vi "DSC TSV to PGSQL.vi"() -> ()   [LabVIEW 2019]
uses:
  src/LV-Data.PG/LV-Data.PGSQL.lvclass
  1022e062-927a-46ce-8191-545f75b782fa.vi
  <vilib>/dlg_ctls.llb/Space Constant.vi
  src/LV-Data.PG/API/Write Variable (multirow).vi
  <vilib>/Utility/error.llb/Clear Errors.vi
  <userlib>/_OpenG.lib/file/file.llb/Build Path - File Names Array__ogtk.vi
  src/LV-Data.PG/Private/INSERT Multivalue.vi
  DSC TSV Process Path.vi
panel:
  in  "Process Files":bool
  in  "Load Translation":bool
  in  "Save Translation":bool
  in  "Get PGSQL":bool
  in  "List Files":bool
  in  "Macro":bool
  out "Status":string
  out "Processed Files":string
  out "Paths":string[][](table)
  in  "Instrument Path":path=path "G:/.shortcut-targets-by-id/1WDr4dR83sFDxMqrJrBnKdnzPXtLPCjmG/Database Data"
  in  "OK":bool
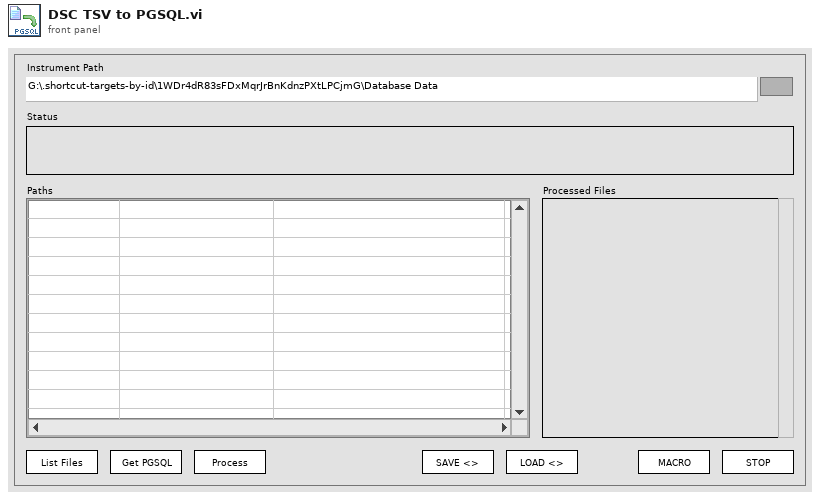
[diagram p1: front panel]
types:
  T1 = enum32{"Invalid", "Standard", "Closed", "Hidden", "Minimized", "Maximized"}
  T2 = enum32{"invalid app kind", "Development System", "Run Time System", "Student Edition", "Embedded LabVIEW", "Evaluation", "Custom"}
  T3 = cluster{"Core":cluster{"Current VI Reference":refnum<vi>, "Close Panel on Exit?":bool}, "Data.PG":refnum<class "LV-Data.PGSQL.lvclass">, "Instrument Path":path, "Variables":path[], "Files":path[][], "DSC Table":string[], "DSC Variable":string[], "DSC Units":string[], "PGSQL Paths":string[]}
  T4 = cluster{"Current VI Reference":refnum<vi>, "Close Panel on Exit?":bool}
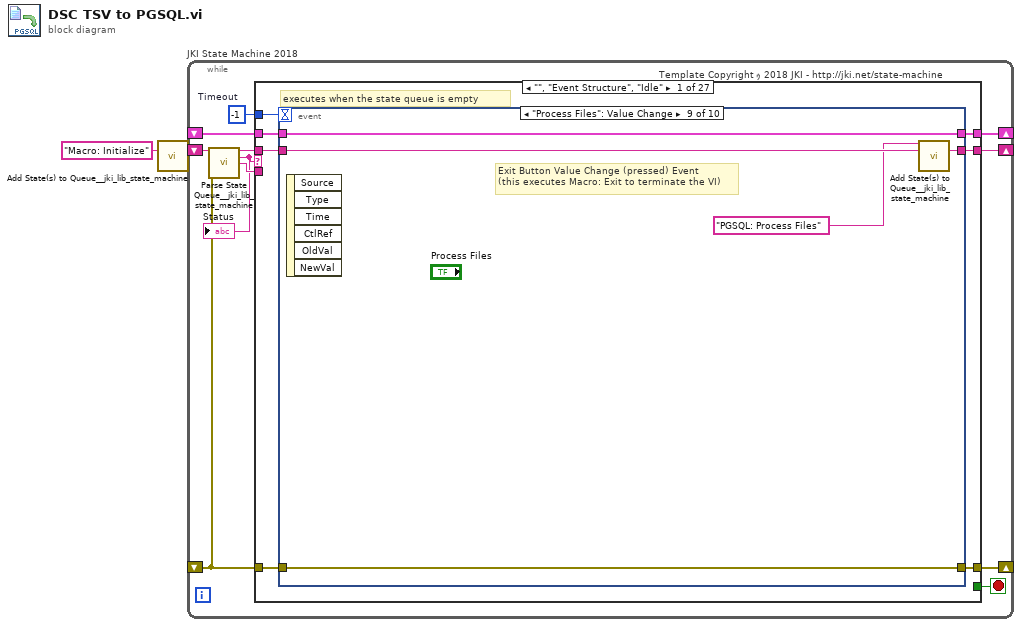
[diagram p0: block diagram]
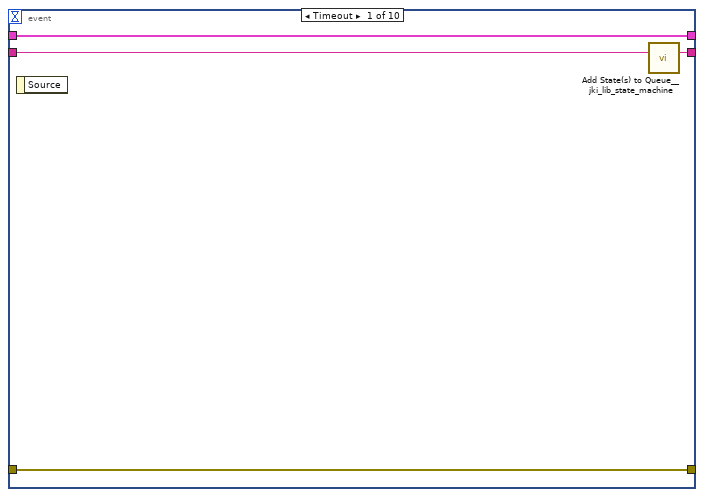
[diagram p2: hidden frame]
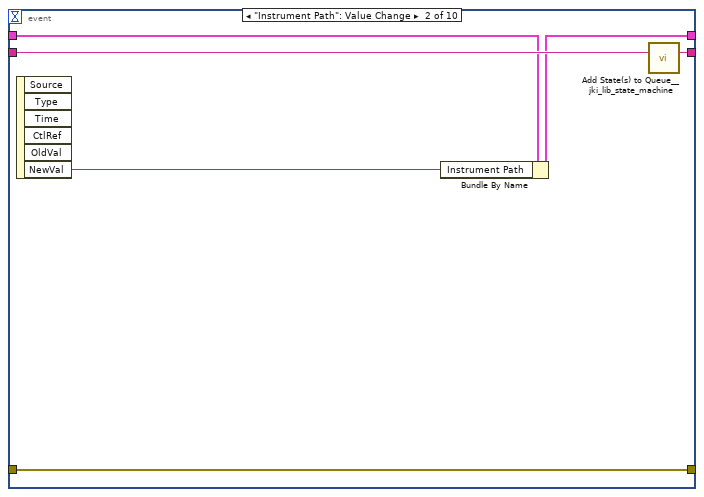
[diagram p3: hidden frame]
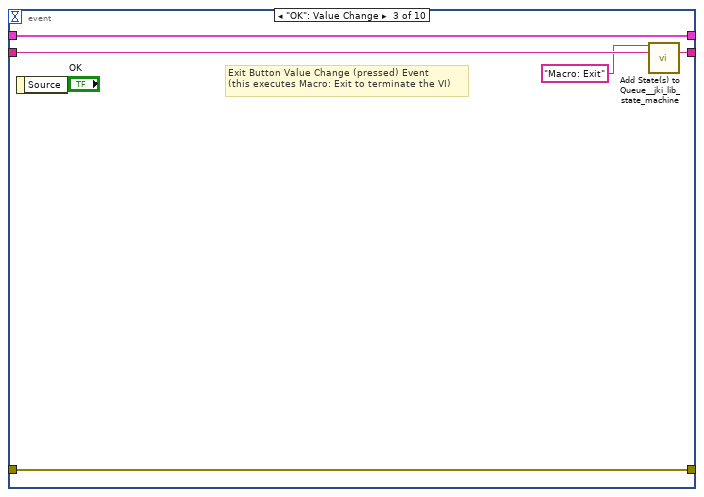
[diagram p4: hidden frame]
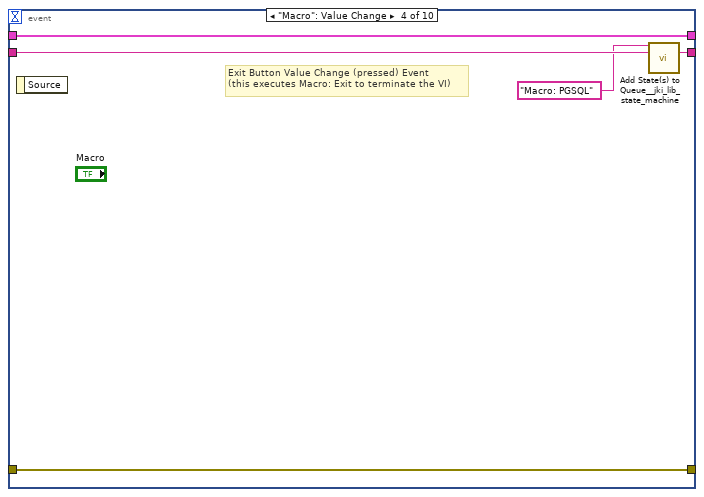
[diagram p5: hidden frame]
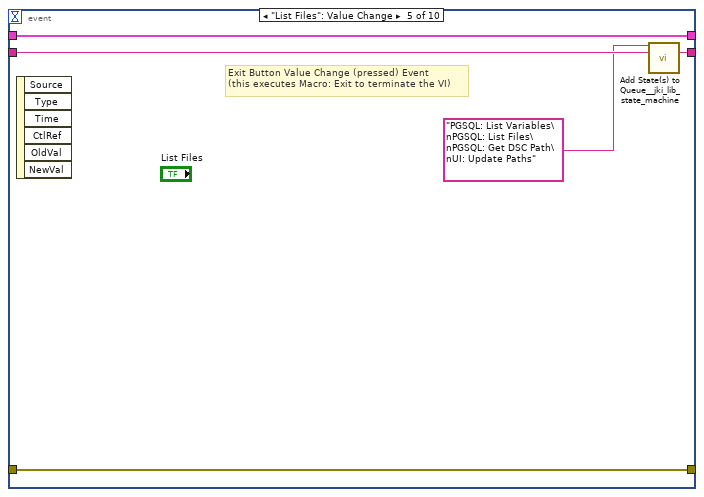
[diagram p6: hidden frame]
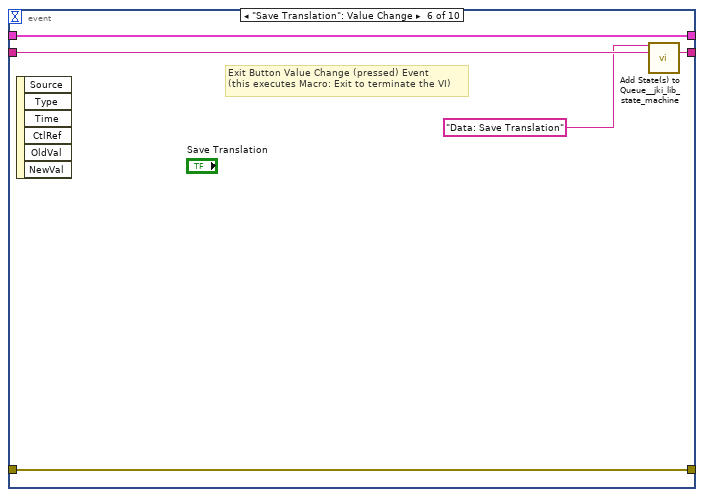
[diagram p7: hidden frame]
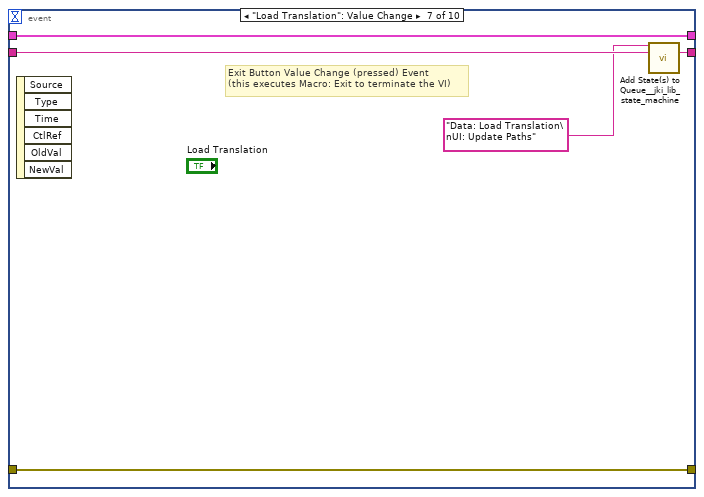
[diagram p8: hidden frame]
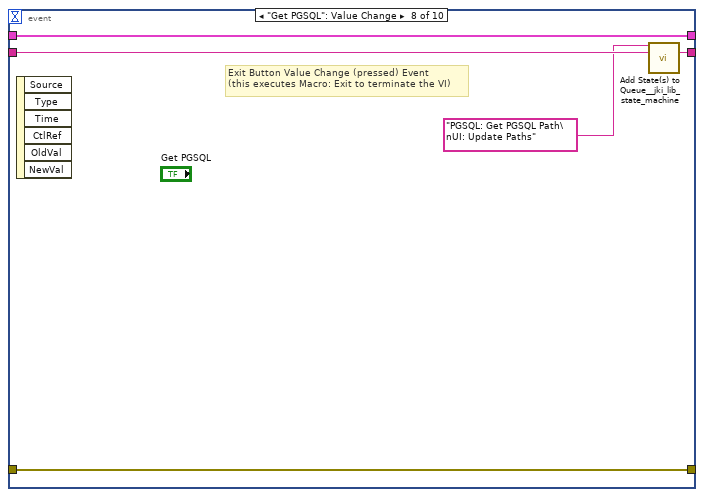
[diagram p9: hidden frame]
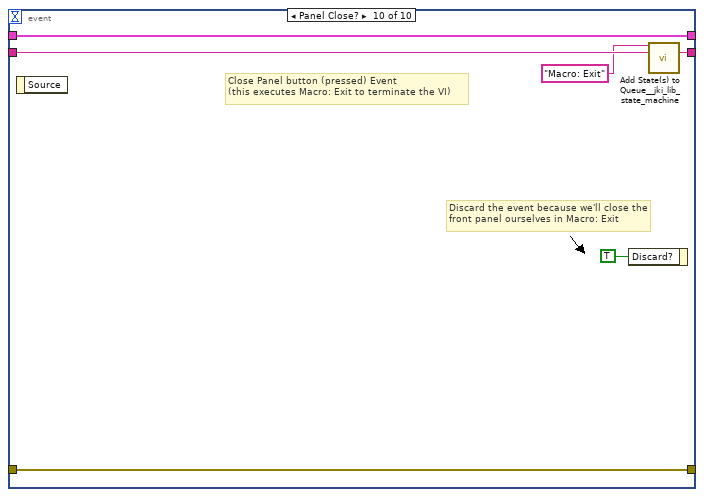
[diagram p10: hidden frame]
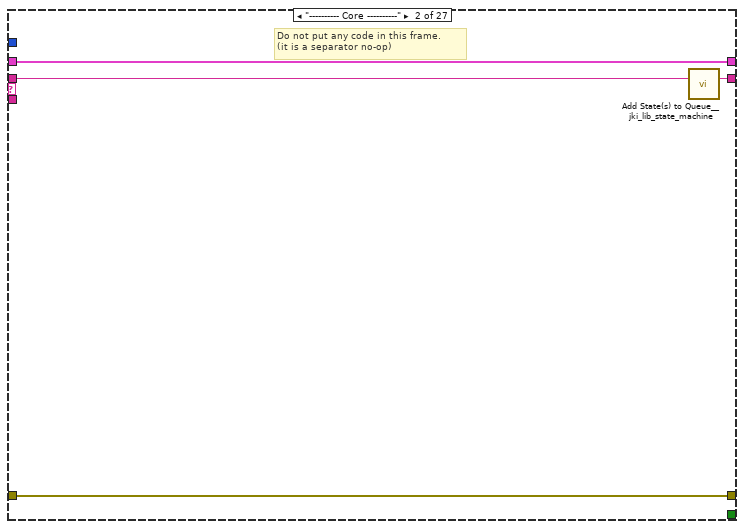
[diagram p11: hidden frame]
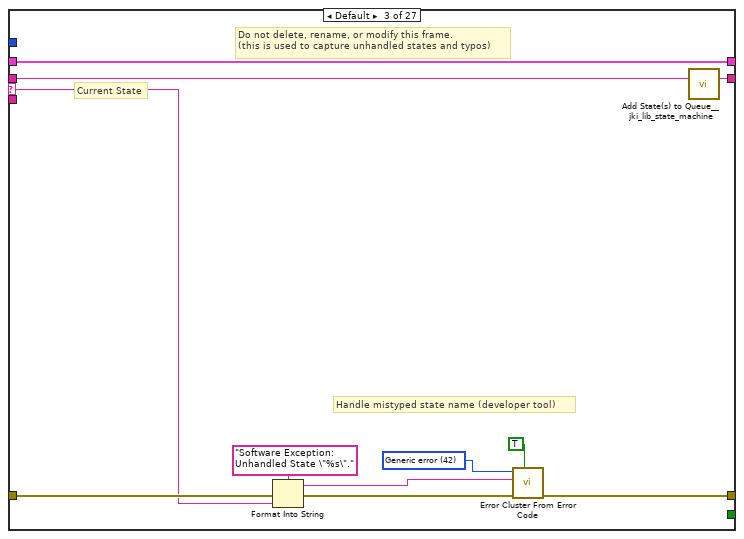
[diagram p12: hidden frame]
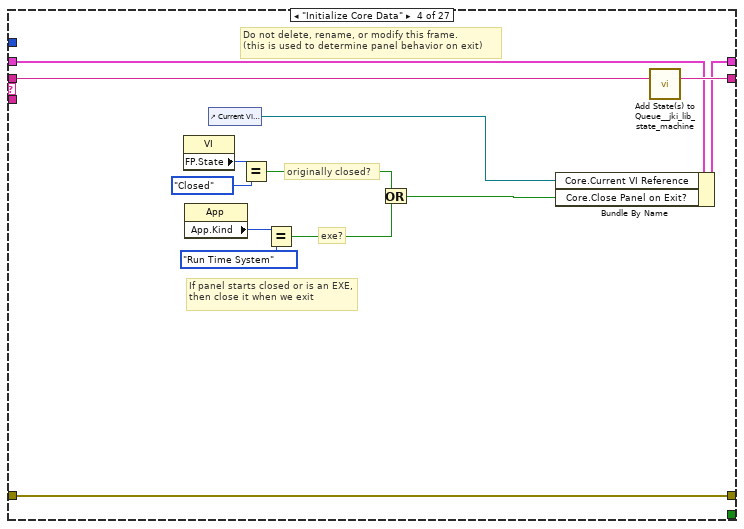
[diagram p13: hidden frame]
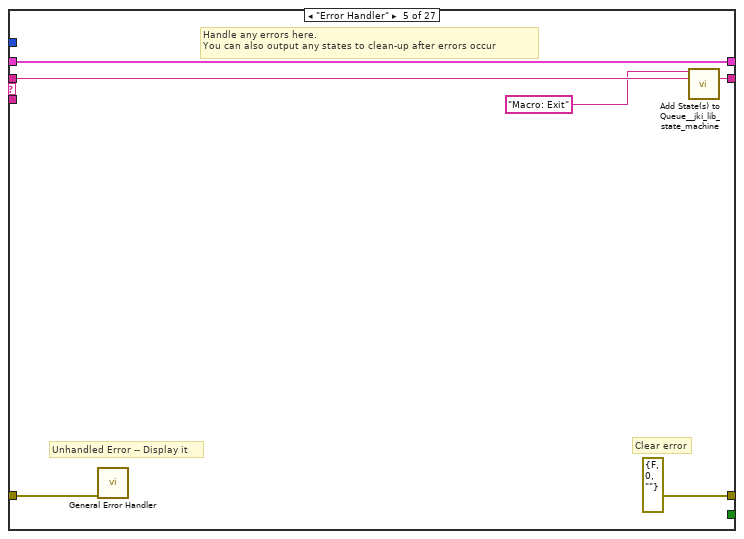
[diagram p14: hidden frame]
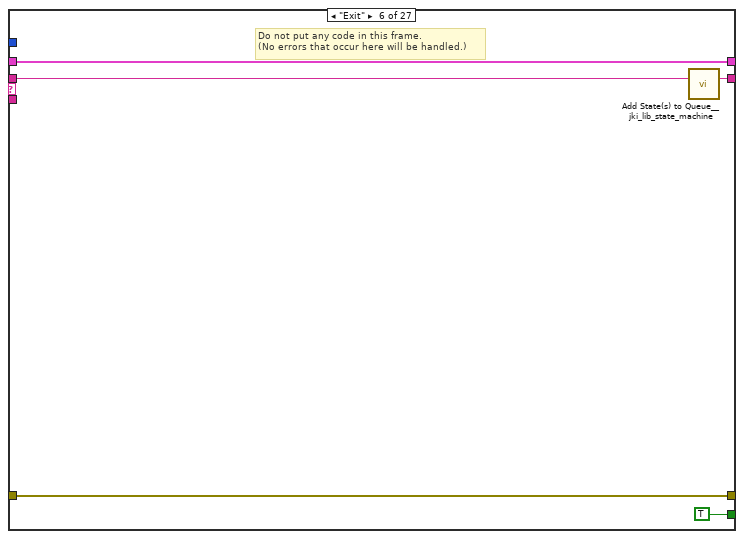
[diagram p15: hidden frame]
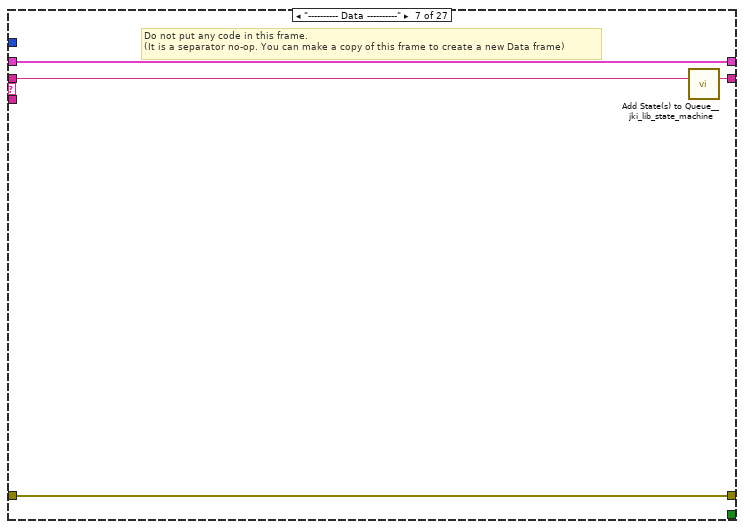
[diagram p16: hidden frame]
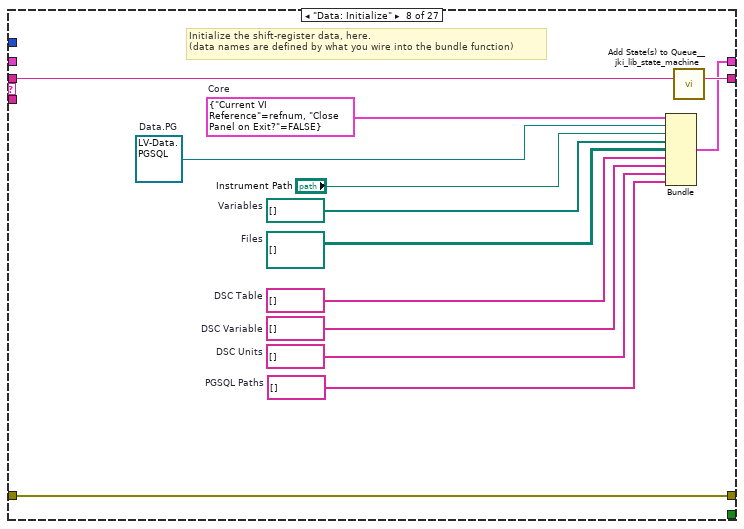
[diagram p17: hidden frame]
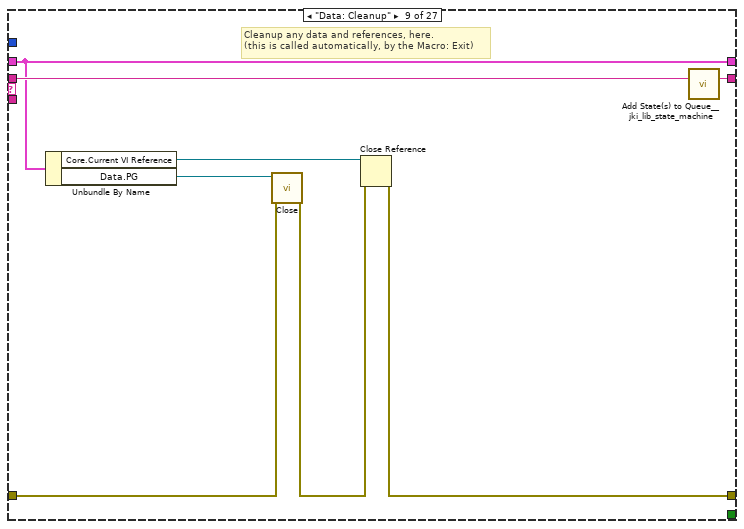
[diagram p18: hidden frame]
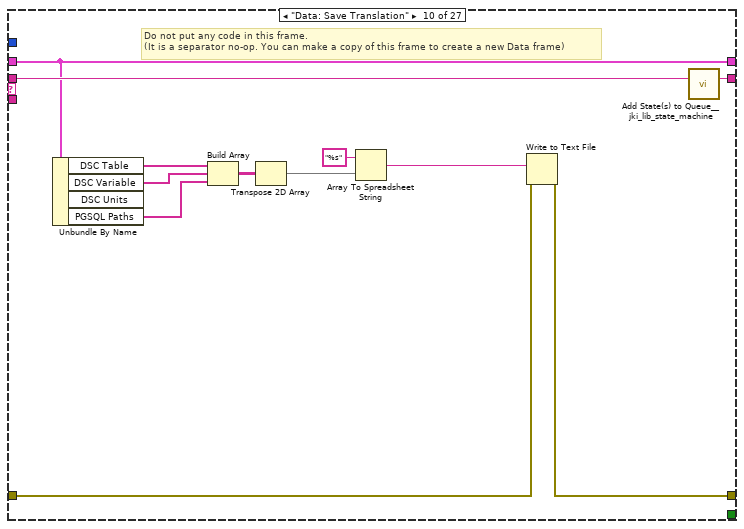
[diagram p19: hidden frame]
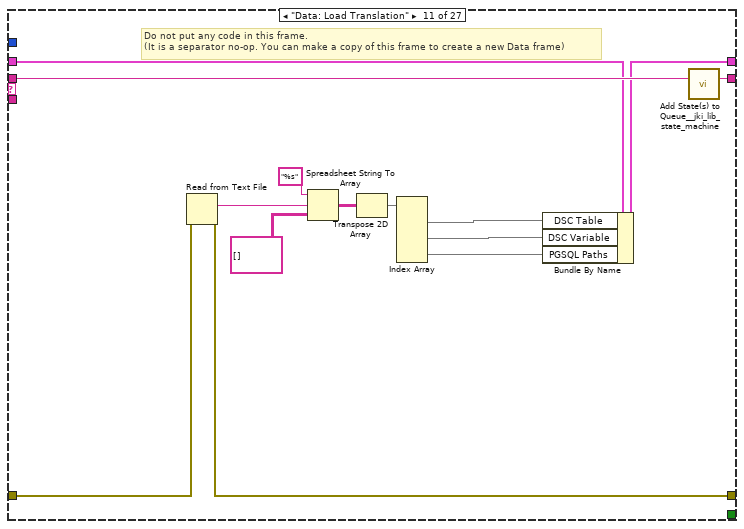
[diagram p20: hidden frame]
diagram:
  n1 = call <vilib>:"Add State(s) to Queue__jki_lib_state_machine.vi"("State(s) in (\"\")"="Macro: Initialize") -> ("States Out"=w2:string)  [unwired: 14 in]
  n2 = while "JKI State Machine 2018" {
    shift-right: [w7] -> _
    shift-left: _ -> [w6]
    shift-right: [w10] -> _
    shift-left: _ -> [w4]
    shift-right: [w9] -> _
    shift-left: w2 -> [w11]
    stop <- w8 stop-if-true
    w5 = -1  # Timeout
    # "Template Copyright ｩ 2018 JKI - http://jki.net/state-machine"
    n3 = call <vilib>:"Parse State Queue__jki_lib_state_machine.vi"("State Queue"=w11, "Error In (no error)"=w4) -> ("Remaining States"=w13:string, "Current State"=w3:string, "Arguments"=w12:string)  [unwired: 11 in]
    "Status" <- w3
    n4 = case shown="\"\", \"Event Structure\", \"Idle\"" w3 {
      selector: w3 -> [_ _ w76 _ _ _ _ _ _ _ _ _ _ _ _ _ _ _ _ _ _ _ _ _ _ _ _]
      tunnel: w13 -> [w20 w75 w80 w99 w105 w110 w114 w127 w135 w147 w161 w165 w169 w175 w193 w200 w269 w274 w279 w289 w293 w301 w310 w319 w349 w391 w430]
      tunnel: w12 -> [_ _ _ _ _ _ _ _ _ _ _ _ _ w170 _ w194 _ _ _ _ _ _ _ _ _ _ _]
      tunnel: w6 -> [w18 w72 w78 w92 w102 w108 w111 _ w131 w142 w151 w162 w167 w173 w190 w196 w266 w271 w276 w286 w290 w296 w302 w311 w339 w386 w428]
      tunnel: [w17 w73 w82 w96 errorcluster {"status"=FALSE, "code"=0, "source"=""} ("error out") w107 w112 w124 w132 w138 w158 w163 w166 w171 w191 w197 w267 w272 w277 w287 w291 w295 w308 w314 w347 w383 w424] -> w10
      tunnel: w4 -> [w16 w73 w81 w96 w101 w107 w112 w124 w128 w137 w159 w163 w166 w172 w191 w198 w267 w272 w277 w287 w291 w294 w308 w315 w347 w384 w425]
      tunnel: [w19 w74 w79 w98 w104 w109 w113 w126 w134 w146 w160 w164 w168 w174 w192 w199 w268 w273 w278 w288 w292 w300 w309 w318 w348 w390 w429] -> w9
      tunnel: [_ _ _ _ _ TRUE _ _ _ _ _ _ _ _ _ _ _ _ _ _ _ _ _ _ _ _ _] -> w8
      tunnel: [w15 w72 w78 w97 w102 w108 w111 w125 w131 w142 w152 w162 w167 w173 w190 w196 w266 w271 w276 w286 w290 w297 w303 w312 w340 w387 w428] -> w7
      tunnel: w5 -> [w14 _ _ _ _ _ _ _ _ _ _ _ _ _ _ _ _ _ _ _ _ _ _ _ _ _ _]
      frame "", "Event Structure", "Idle" {
        # "executes when the state queue is empty"
        n5 = event shown="[8] \"Process Files\": Value Change" {
          selector: _ -> [_ _ _ _ _ _ _ _ _ _]
          dyn-events: _ -> [_ _ _ _ _ _ _ _ _ _]
          timeout: w14 -> [_ _ _ _ _ _ _ _ _ _]
          tunnel: w20 -> [w24 w30 w35 w40 w45 w50 w55 w60 w65 w71]
          tunnel: [w23 w29 w34 w39 w44 w49 w54 w59 w64 w70] -> w19
          tunnel: w18 -> [w21 w25 w32 w37 w42 w47 w52 w57 w62 w68]
          tunnel: [w22 w28 w33 w38 w43 w48 w53 w58 w63 w69] -> w17
          tunnel: w16 -> [w22 w28 w33 w38 w43 w48 w53 w58 w63 w69]
          tunnel: [w21 w26 w32 w37 w42 w47 w52 w57 w62 w68] -> w15
          event Timeout {
            n6 = event-data() -> ()  [unwired: 1 in, 1 out]
            n7 = call <vilib>:"Add State(s) to Queue__jki_lib_state_machine.vi"("State(s) in (\"\")"=w24) -> ("States Out"=w23:string)  [unwired: 14 in]
          }
          event "Instrument Path": Value Change {
            n8 = event-data() -> ("NewVal"=w27:path)  [unwired: 1 in, 5 out]
            n9 = Bundle By Name(cluster=w25, "Instrument Path"=w27) -> (w26:T3)
            n10 = call <vilib>:"Add State(s) to Queue__jki_lib_state_machine.vi"("State(s) in (\"\")"=w30) -> ("States Out"=w29:string)  [unwired: 14 in]
          }
          event "OK": Value Change {
            # "Exit Button Value Change (pressed) Event\n(this executes Macro: Exit to terminate the VI)"
            n11 = event-data() -> ()  [unwired: 1 in, 1 out]
            n12 = call <vilib>:"Add State(s) to Queue__jki_lib_state_machine.vi"("State(s) in Front (\"\")"="Macro: Exit", "State(s) in (\"\")"=w35) -> ("States Out"=w34:string)  [unwired: 13 in]
          }
          event "Macro": Value Change {
            # "Exit Button Value Change (pressed) Event\n(this executes Macro: Exit to terminate the VI)"
            n13 = event-data() -> ()  [unwired: 1 in, 1 out]
            n14 = call <vilib>:"Add State(s) to Queue__jki_lib_state_machine.vi"("State(s) in Front (\"\")"="Macro: PGSQL", "State(s) in (\"\")"=w40) -> ("States Out"=w39:string)  [unwired: 13 in]
          }
          event "List Files": Value Change {
            # "Exit Button Value Change (pressed) Event\n(this executes Macro: Exit to terminate the VI)"
            n15 = event-data() -> ()  [unwired: 1 in, 6 out]
            n16 = call <vilib>:"Add State(s) to Queue__jki_lib_state_machine.vi"("State(s) in Front (\"\")"="PGSQL: List Variables\nPGSQL: List Files\nPGSQL: Get DSC Path\nUI: Update Paths", "State(s) in (\"\")"=w45) -> ("States Out"=w44:string)  [unwired: 13 in]
          }
          event "Save Translation": Value Change {
            # "Exit Button Value Change (pressed) Event\n(this executes Macro: Exit to terminate the VI)"
            n17 = event-data() -> ()  [unwired: 1 in, 6 out]
            n18 = call <vilib>:"Add State(s) to Queue__jki_lib_state_machine.vi"("State(s) in Front (\"\")"="Data: Save Translation", "State(s) in (\"\")"=w50) -> ("States Out"=w49:string)  [unwired: 13 in]
          }
          event "Load Translation": Value Change {
            # "Exit Button Value Change (pressed) Event\n(this executes Macro: Exit to terminate the VI)"
            n19 = event-data() -> ()  [unwired: 1 in, 6 out]
            n20 = call <vilib>:"Add State(s) to Queue__jki_lib_state_machine.vi"("State(s) in Front (\"\")"="Data: Load Translation\nUI: Update Paths", "State(s) in (\"\")"=w55) -> ("States Out"=w54:string)  [unwired: 13 in]
          }
          event "Get PGSQL": Value Change {
            # "Exit Button Value Change (pressed) Event\n(this executes Macro: Exit to terminate the VI)"
            n21 = event-data() -> ()  [unwired: 1 in, 6 out]
            n22 = call <vilib>:"Add State(s) to Queue__jki_lib_state_machine.vi"("State(s) in Front (\"\")"="PGSQL: Get PGSQL Path\nUI: Update Paths", "State(s) in (\"\")"=w60) -> ("States Out"=w59:string)  [unwired: 13 in]
          }
          event "Process Files": Value Change {
            # "Exit Button Value Change (pressed) Event\n(this executes Macro: Exit to terminate the VI)"
            n23 = event-data() -> ()  [unwired: 1 in, 6 out]
            n24 = call <vilib>:"Add State(s) to Queue__jki_lib_state_machine.vi"("State(s) in Front (\"\")"="PGSQL: Process Files", "State(s) in (\"\")"=w65) -> ("States Out"=w64:string)  [unwired: 13 in]
          }
          event Panel Close? {
            # "Discard the event because we'll close the front panel ourselves in Macro: Exit"
            # "Close Panel button (pressed) Event\n(this executes Macro: Exit to terminate the VI)"
            n25 = event-data() -> ()  [unwired: 1 in, 1 out]
            n26 = event-data("Discard?"=TRUE) -> ()  [unwired: 1 in, 1 out]
            n27 = call <vilib>:"Add State(s) to Queue__jki_lib_state_machine.vi"("State(s) in Front (\"\")"="Macro: Exit", "State(s) in (\"\")"=w71) -> ("States Out"=w70:string)  [unwired: 13 in]
          }
        }
      }
      frame "---------- Core ----------" {
        # "Do not put any code in this frame.\n(it is a separator no-op)"
        n28 = call <vilib>:"Add State(s) to Queue__jki_lib_state_machine.vi"("State(s) in (\"\")"=w75) -> ("States Out"=w74:string)  [unwired: 14 in]
      }
      frame Default {
        w85 = 42 items=["No error", "Argument error", "Memory is full", "Out of zone", "End of file", "File already open", "Generic file I/O error", "File not found", "File permission error", "Disk is full", "Duplicate path", "Too many files open", "System feature not enabled", "Resource file not found", "Cannot add resource", "Resource not found", "Image not found", "Image memory error", "Pen does not exist", "Config type invalid", "Config token not found", "Config parse error", "Config memory error", "Bad external code format", "Bad external code offset", "External code not present", "Null window", "Destroy window error", "Null menu", "Print aborted", "Bad print record", "Print driver error", "Windows error during printing", "Memory error during printing", "Print dialog error", "Generic print error", "Invalid device refnum", "Device not found", "Device parameter error", "Device unit error", "Cannot open device", "Device call aborted", "Generic error", "Cancelled by user", "Object ID too low", "Object ID too high", "Object not in heap", "Unknown heap", "Unknown object (invalid DefProc)", "Unknown object (DefProc not in table)", "Message out of range", "Invalid (null) method", "Unknown message", "Manager call not supported", "Bad address", "Network operation in progress", "Network operation timed out", "Connection is busy", "Network attribute not supported", "Network error", "Address in use", "System out of memory", "Connection aborted", "Connection refused", "Not connected", "Already connected", "Connection closed", "Initialization error (interapplication manager)", "Bad occurrence", "Wait on unbound occurrence handler", "Occurrence queue overflow", "Datalog type conflict", "Unused", "Unrecognized type (interapplication manager)", "Memory corrupt", "Failed to make temporary DLL", "Old CIN version", "Drag socket not found", "Failed to load drop-object", "Failed to register OLE object", "Failed to release OLE object", "Format specifier type mismatch", "Unknown format specifier", "Too few format specifiers", "Too many format specifiers", "Scan failed", "Newer CIN version", "Error converting to variant", "Runtime menu error", "Password tampered", "Variant attribute not found", "Incompatible variant data type", "Event data is not available", "Event Store is not present", "Occurrence is not found", "Event Queue is not created", "Event info is not available", "Refnum passed is NULL", "Error retrieving Class GUID", "Error retrieving CoClass GUID", "Error retrieving TypeLib GUID.", "Bad built application magic bytes.", "Specific driver is different from the specific driver associated with the Logical Name.", "There is no session opened to the class driver.", "Max Error", "MAX - Error with config objects", "MAX - Error loading configuration", "MAX - Group not supported"]
        # "Current State"
        # "Do not delete, rename, or modify this frame.\n(this is used to capture unhandled states and typos)"
        # "Handle mistyped state name (developer tool)"
        n29 = Format Into String(format string="Software Exception: Unhandled State \"%s\"." ("message"), error in=w81, w76) -> (resulting string=w84:string, error out=w83:errorcluster)  [unwired: 1 in]
        n30 = call <vilib>:"Error Cluster From Error Code.vi"("show call chain? (False)"=TRUE, "error in (no error)"=w83, "error message (\"\")"=w84, "error code (0)"=w85) -> ("error out"=w82:errorcluster)  [unwired: 5 in]
        n31 = call <vilib>:"Add State(s) to Queue__jki_lib_state_machine.vi"("State(s) in (\"\")"=w80) -> ("States Out"=w79:string)  [unwired: 14 in]
      }
      frame "Initialize Core Data" {
        # "Do not delete, rename, or modify this frame.\n(this is used to determine panel behavior on exit)"
        # "originally closed?"
        # "exe?"
        # "If panel starts closed or is an EXE, then close it when we exit"
        n32 = property class="VI"() -> ("FP.State"=w89:T1)  [unwired: 2 in, 2 out]
        n33 = property class="App"() -> ("App.Kind"=w95:T2)  [unwired: 2 in, 2 out]
        n34 = control-ref of="Current VI Reference"() -> (w90:refnum<vi>)
        n35 = Equal?(x=w89, y=T1."Closed" ("Front Panel Window:State")) -> (x = y?=w87:bool)
        n36 = Equal?(x=w95, y=T2."Run Time System" ("Application:Kind")) -> (x = y?=w93:bool)
        n37 = Or(x=w87, y=w93) -> (x .or. y?=w91:bool)
        n38 = Bundle By Name(cluster=w92, "Core.Current VI Reference"=w90, "Core.Close Panel on Exit?"=w91) -> (w97:T3)
        n39 = call <vilib>:"Add State(s) to Queue__jki_lib_state_machine.vi"("State(s) in (\"\")"=w99) -> ("States Out"=w98:string)  [unwired: 14 in]
      }
      frame "Error Handler" {
        # "Unhandled Error -- Display it"
        # "Handle any errors here.\nYou can also output any states to clean-up after errors occur"
        # "Clear error"
        n40 = call <vilib>:"General Error Handler.vi"("error in (no error)"=w101) -> ()  [unwired: 10 in, 5 out]
        n41 = call <vilib>:"Add State(s) to Queue__jki_lib_state_machine.vi"("State(s) in Front (\"\")"="Macro: Exit", "State(s) in (\"\")"=w105) -> ("States Out"=w104:string)  [unwired: 13 in]
      }
      frame "Exit" {
        # "Do not put any code in this frame.\n(No errors that occur here will be handled.)"
        n42 = call <vilib>:"Add State(s) to Queue__jki_lib_state_machine.vi"("State(s) in (\"\")"=w110) -> ("States Out"=w109:string)  [unwired: 14 in]
      }
      frame "---------- Data ----------" {
        # "Do not put any code in this frame.\n(It is a separator no-op. You can make a copy of this frame to create a new Data frame)"
        n43 = call <vilib>:"Add State(s) to Queue__jki_lib_state_machine.vi"("State(s) in (\"\")"=w114) -> ("States Out"=w113:string)  [unwired: 14 in]
      }
      frame "Data: Initialize" {
        w115 = refnum<class "LV-Data.PGSQL.lvclass"> refnum  # Data.PG
        w116 = string[] []  # PGSQL Paths
        w117 = string[] []  # DSC Units
        w118 = string[] []  # DSC Variable
        w119 = string[] []  # DSC Table
        w121 = path[] []  # Variables
        w120 = path[][] []  # Files
        w123 = T4 {"Current VI Reference"=refnum, "Close Panel on Exit?"=FALSE}  # Core
        # "Initialize the shift-register data, here.\n(data names are defined by what you wire into the bundle function)"
        n44 = Bundle("Core"=w123, "Data.PG"=w115, "Instrument Path"="Instrument Path", "Variables"=w121, "Files"=w120, "DSC Table"=w119, "DSC Variable"=w118, "DSC Units"=w117, "PGSQL Paths"=w116) -> (w125:T3)  [unwired: 1 in]
        n45 = call <vilib>:"Add State(s) to Queue__jki_lib_state_machine.vi"("State(s) in (\"\")"=w127) -> ("States Out"=w126:string)  [unwired: 14 in]
      }
      frame "Data: Cleanup" {
        # "Cleanup any data and references, here.\n(this is called automatically, by the Macro: Exit)"
        n46 = Unbundle By Name(w131) -> ("Core.Current VI Reference"=w133:refnum<vi>, "Data.PG"=w130:refnum<class "LV-Data.PGSQL.lvclass">)
        n47 = call-dynamic "Close.vi"("error in (no error)"=w128, "Data.PG in"=w130) -> ("error out"=w129:errorcluster)  [unwired: 8 in, 1 out]
        n48 = Close Reference(reference=w133, error in (no error)=w129) -> (error out=w132:errorcluster)
        n49 = call <vilib>:"Add State(s) to Queue__jki_lib_state_machine.vi"("State(s) in (\"\")"=w135) -> ("States Out"=w134:string)  [unwired: 14 in]
      }
      frame "Data: Save Translation" {
        # "Do not put any code in this frame.\n(It is a separator no-op. You can make a copy of this frame to create a new Data frame)"
        n50 = Unbundle By Name(w142) -> ("DSC Table"=w145:string[], "DSC Variable"=w143:string[], "PGSQL Paths"=w144:string[])  [unwired: 1 out]
        n51 = Build Array(w145, w143, w144) -> (w141:string[][])
        n52 = Transpose 2D Array(2D array=w141) -> (transposed array=w136:string[][])
        n53 = Array To Spreadsheet String(array=w136, 3:"%s" ("format string")) -> (spreadsheet string=w139:string)  [unwired: 1 in]
        n54 = Write to Text File(text=w139, error in=w137) -> (error out=w138:errorcluster)  [unwired: 2 in, 2 out]
        n55 = call <vilib>:"Add State(s) to Queue__jki_lib_state_machine.vi"("State(s) in (\"\")"=w147) -> ("States Out"=w146:string)  [unwired: 14 in]
      }
      frame "Data: Load Translation" {
        # "Do not put any code in this frame.\n(It is a separator no-op. You can make a copy of this frame to create a new Data frame)"
        n56 = Read from Text File(error in=w159) -> (text=w150:string, error out=w158:errorcluster)  [unwired: 3 in, 2 out]
        n57 = Spreadsheet String To Array(format string="%s", spreadsheet string=w150, array type (2D Dbl)=string[][] [] ("appended array")) -> (array=w157:string[][])  [unwired: 1 in]
        n58 = Transpose 2D Array(2D array=w157) -> (transposed array=w148:string[][])
        n59 = Index Array(array=w148) -> (element #1=w153:string[], element #2=w154:string[], element #3=w155:string[])  [unwired: 6 in]
        n60 = Bundle By Name(cluster=w151, "DSC Table"=w153, "DSC Variable"=w154, "PGSQL Paths"=w155) -> (w152:T3)
        n61 = call <vilib>:"Add State(s) to Queue__jki_lib_state_machine.vi"("State(s) in (\"\")"=w161) -> ("States Out"=w160:string)  [unwired: 14 in]
      }
      frame "---------- UI ----------" {
        # "Do not put any code in this frame.\n(It is a separator no-op. You can make a copy of this frame to create a new UI frame)"
        n62 = call <vilib>:"Add State(s) to Queue__jki_lib_state_machine.vi"("State(s) in (\"\")"=w165) -> ("States Out"=w164:string)  [unwired: 14 in]
      }
      frame "UI: Initialize" {
        # "Initialize the User Interface, here.\n(this is called automatically, by the Macro: Init)"
        n63 = invoke on="Processed Files" class="Str" method="Reinit To Default"() -> ()  [unwired: 3 in, 3 out]
        n64 = invoke on="Paths" class="Tbl (strict)" method="Reinit To Default"() -> ()  [unwired: 3 in, 3 out]
        n65 = call <userlib>:"Fit VI window to Largest Dec__ogtk.vi"() -> ()  [unwired: 6 in, 2 out]
        n66 = call <vilib>:"Add State(s) to Queue__jki_lib_state_machine.vi"("State(s) in (\"\")"=w169) -> ("States Out"=w168:string)  [unwired: 14 in]
      }
      frame "UI: Cursor Set" {
        # "Argument"
        # "Set and Unset Cursor Busy.\n(Usage: \"UI: Cursor Set >> Busy|Idle\")"
        n67 = case shown="\"Busy\"" w170 {
          tunnel: w172 -> [w177 w179]
          tunnel: [w176 w178] -> w171
          frame "Idle", Default {
            n68 = call <vilib>:"Unset Busy.vi"("error in (no error)"=w177) -> ("error out"=w176:errorcluster)  [unwired: 10 in]
          }
          frame "Busy" {
            n69 = call <vilib>:"Set Busy.vi"("error in (no error)"=w179) -> ("error out"=w178:errorcluster)  [unwired: 9 in, 1 out]
          }
        }
        n70 = call <vilib>:"Add State(s) to Queue__jki_lib_state_machine.vi"("State(s) in (\"\")"=w175) -> ("States Out"=w174:string)  [unwired: 14 in]
      }
      frame "UI: Update Paths" {
        # "Do not put any code in this frame.\n(It is a separator no-op. You can make a copy of this frame to create a new UI frame)"
        n71 = Unbundle By Name(w190) -> ("DSC Table"=w189:string[], "DSC Variable"=w187:string[], "PGSQL Paths"=w188:string[])  [unwired: 1 out]
        n72 = Build Array(w189, w187, w188) -> (w183:string[][])
        n73 = Build Array("DSC Table" ("format string"), "DSC Variable" ("format string"), "PGSQL Path" ("format string")) -> (w181:string[])
        n74 = Transpose 2D Array(2D array=w183) -> (transposed array=w182:string[][])
        n75 = Build Array (concatenate)(w181, w182) -> (→"Paths":string[][])
        n76 = call <vilib>:"Add State(s) to Queue__jki_lib_state_machine.vi"("State(s) in (\"\")"=w193) -> ("States Out"=w192:string)  [unwired: 14 in]
      }
      frame "UI: Front Panel State" {
        # "Argument"
        # "Set Front Panel Open or Closed\n(Usage: \"UI: Front Panel State >> Open|Close\")"
        n77 = Unbundle By Name(w196) -> ("Core.Current VI Reference"=w195:refnum<vi>)
        n78 = case shown="\"Minimize\", \"Minimized\"" w194 {
          tunnel: w198 -> [w206 w221 w232 w245 w258]
          tunnel: [w208 w222 w234 w247 w260] -> w197
          tunnel: w195 -> [w207 w219 w233 w246 w259]
          frame "Open", "Standard", Default {
            w201 = T1."Standard" ("State")
            n79 = property class="VI"(reference=w207, error in=w206) -> (reference out=w204:refnum<vi>, error out=w205:errorcluster, "FP.State"=w203:T1)
            n80 = Not Equal?(x=w203, y=w201) -> (x != y?=w202:bool)
            n81 = case shown="True" w202 {
              tunnel: [w212 w214] -> w208
              tunnel: w205 -> [w211 w214]
              tunnel: w204 -> [w210 _]
              tunnel: w201 -> [w209 _]
              frame True {
                n82 = invoke class="VI" method="FP.Open"(reference=w210, error in=w211, "Activate"=TRUE, "State"=w209) -> (error out=w212:errorcluster)  [unwired: 1 in, 4 out]
              }
              frame False {
              }
            }
          }
          frame "Close", "Closed" {
            n83 = property class="VI"(reference=w219, error in=w221) -> (reference out=w218:refnum<vi>, error out=w220:errorcluster, "FP.State"=w216:T1)
            n84 = Not Equal?(x=w216, y=T1."Closed" ("Front Panel Window:State")) -> (x != y?=w215:bool)
            n85 = case shown="True" w215 {
              tunnel: [w223 w226] -> w222
              tunnel: w220 -> [w223 w225]
              tunnel: w218 -> [_ w224]
              frame False {
              }
              frame True {
                n86 = invoke class="VI" method="FP.Close"(reference=w224, error in=w225) -> (error out=w226:errorcluster)  [unwired: 1 in, 2 out]
              }
            }
          }
          frame "Hidden", "Hide" {
            w227 = T1."Hidden" ("State")
            n87 = property class="VI"(reference=w233, error in=w232) -> (reference out=w230:refnum<vi>, error out=w231:errorcluster, "FP.State"=w229:T1)
            n88 = Not Equal?(x=w229, y=w227) -> (x != y?=w228:bool)
            n89 = case shown="True" w228 {
              tunnel: [w238 w239] -> w234
              tunnel: w231 -> [w237 w239]
              tunnel: w230 -> [w236 _]
              tunnel: w227 -> [w235 _]
              frame True {
                n90 = invoke class="VI" method="FP.Open"(reference=w236, error in=w237, "State"=w235) -> (error out=w238:errorcluster)  [unwired: 2 in, 4 out]
              }
              frame False {
              }
            }
          }
          frame "Minimize", "Minimized" {
            w240 = T1."Minimized" ("State")
            n91 = property class="VI"(reference=w246, error in=w245) -> (reference out=w243:refnum<vi>, error out=w244:errorcluster, "FP.State"=w242:T1)
            n92 = Not Equal?(x=w242, y=w240) -> (x != y?=w241:bool)
            n93 = case shown="True" w241 {
              tunnel: [w251 w252] -> w247
              tunnel: w244 -> [w250 w252]
              tunnel: w243 -> [w249 _]
              tunnel: w240 -> [w248 _]
              frame True {
                n94 = invoke class="VI" method="FP.Open"(reference=w249, error in=w250, "State"=w248) -> (error out=w251:errorcluster)  [unwired: 2 in, 4 out]
              }
              frame False {
              }
            }
          }
          frame "Maximize", "Maximized" {
            w253 = T1."Maximized" ("State")
            n95 = property class="VI"(reference=w259, error in=w258) -> (reference out=w256:refnum<vi>, error out=w257:errorcluster, "FP.State"=w255:T1)
            n96 = Not Equal?(x=w255, y=w253) -> (x != y?=w254:bool)
            n97 = case shown="True" w254 {
              tunnel: [w264 w265] -> w260
              tunnel: w257 -> [w263 w265]
              tunnel: w256 -> [w262 _]
              tunnel: w253 -> [w261 _]
              frame True {
                n98 = invoke class="VI" method="FP.Open"(reference=w262, error in=w263, "State"=w261) -> (error out=w264:errorcluster)  [unwired: 2 in, 4 out]
              }
              frame False {
              }
            }
          }
        }
        n99 = call <vilib>:"Add State(s) to Queue__jki_lib_state_machine.vi"("State(s) in (\"\")"=w200) -> ("States Out"=w199:string)  [unwired: 14 in]
      }
      frame "---------- Macro ----------" {
        # "Do not put any code in this frame.\n(It is a separator no-op. You can make a copy of this frame to create a new Macro frame)"
        n100 = call <vilib>:"Add State(s) to Queue__jki_lib_state_machine.vi"("State(s) in (\"\")"=w269) -> ("States Out"=w268:string)  [unwired: 14 in]
      }
      frame "Macro: Initialize" {
        w270 = "Data: Initialize\nInitialize Core Data\nUI: Initialize\nUI: Front Panel State >> Open\nPGSQL: Open"  # Data: Initialize Initialize Core Data UI: Initialize UI: Front Panel State >> Open PGSQL: Open
        # "Initialization Macro\n(This is called once, when the VI starts)"
        n101 = call <vilib>:"Add State(s) to Queue__jki_lib_state_machine.vi"("State(s) in Front (\"\")"=w270, "State(s) in (\"\")"=w274) -> ("States Out"=w273:string)  [unwired: 13 in]
      }
      frame "Macro: PGSQL" {
        # "Do not put any code in this frame.\n(It is a separator no-op. You can make a copy of this frame to create a new Macro frame)"
        n102 = call <vilib>:"Add State(s) to Queue__jki_lib_state_machine.vi"("State(s) in Front (\"\")"="PGSQL: List Variables\nPGSQL: List Files\nPGSQL: Get DSC Path\nUI: Update Paths\n//PGSQL: Get PGSQL Path\n// UI: Update Paths\n//PGSQL: Process Files" ("State(s) in Front (\"\")"), "State(s) in (\"\")"=w279) -> ("States Out"=w278:string)  [unwired: 13 in]
      }
      frame "Macro: Exit" {
        # "Exit Macro\n(This is called once, when the VI exits)"
        n103 = Unbundle By Name(w286) -> ("Core.Close Panel on Exit?"=w285:bool)
        n104 = Select(t="UI: Front Panel State >> Close", s=w285, f="") -> (s? t:f=w282:string)
        n105 = call <vilib>:"Add State(s) to Queue__jki_lib_state_machine.vi"("State(s) in (\"\")"=w282, "State(s) at Back (\"\")"="Data: Cleanup\nExit") -> ("States Out"=w280:string)  [unwired: 13 in]
        n106 = call <vilib>:"Add State(s) to Queue__jki_lib_state_machine.vi"("State(s) in Front (\"\")"=w280, "State(s) in (\"\")"=w289) -> ("States Out"=w288:string)  [unwired: 13 in]
      }
      frame "---------- PGSQL ----------" {
        # "Template Separator\n(You can make a copy of, or modify, this frame)"
        n107 = call <vilib>:"Add State(s) to Queue__jki_lib_state_machine.vi"("State(s) in (\"\")"=w293) -> ("States Out"=w292:string)  [unwired: 14 in]
      }
      frame "PGSQL: Open" {
        # "Template Separator\n(You can make a copy of, or modify, this frame)"
        n108 = Unbundle By Name(w296) -> ("Data.PG"=w299:refnum<class "LV-Data.PGSQL.lvclass">)
        n109 = call-dynamic "Open.vi"("error in (no error)"=w294, "Data in"=w299) -> ("error out"=w295:errorcluster, "Data out"=w298:refnum<class "LV-Data.PGSQL.lvclass">)  [unwired: 8 in]
        n110 = Bundle By Name(cluster=w296, "Data.PG"=w298) -> (w297:T3)
        n111 = call <vilib>:"Add State(s) to Queue__jki_lib_state_machine.vi"("State(s) in (\"\")"=w301) -> ("States Out"=w300:string)  [unwired: 14 in]
      }
      frame "PGSQL: List Variables" {
        # "Your code here.\n(You can make a copy of, or modify, this frame)"
        n112 = Unbundle By Name(w302) -> ("Instrument Path"=w305:path)
        n113 = List Folder(path=w305) -> (path out=w306:path, folder names=w307:string[])  [unwired: 3 in, 2 out]
        n114 = call-poly <userlib>:"Build Path__ogtk.vi"("name or relative path"=w307, "base path"=w306) -> ("appended path"=w304:path[])
        n115 = Bundle By Name(cluster=w302, "Variables"=w304) -> (w303:T3)
        n116 = call <vilib>:"Add State(s) to Queue__jki_lib_state_machine.vi"("State(s) in (\"\")"=w310) -> ("States Out"=w309:string)  [unwired: 14 in]
      }
      frame "PGSQL: List Files" {
        # "Your code here.\n(You can make a copy of, or modify, this frame)"
        n117 = Unbundle By Name(w311) -> ("Variables"=w317:path[])
        n118 = for {
          tunnel: w317 -> [w324] mode=indexing
          tunnel: w315 -> [w322]
          tunnel: [w327] -> w316 mode=indexing
          tunnel: [w326] -> w313 mode=indexing
          n119 = Format Into String(format string="Listing %s", error in=w322, w324) -> (resulting string=w325:string, error out=w323:errorcluster)  [unwired: 1 in]
          n120 = local write "Status"(w325) -> ()
          n121 = List Folder(path=w324, error in=w323) -> (path out=w331:path, filenames=w330:string[], error out=w321:errorcluster)  [unwired: 2 in, 1 out]
          n122 = call-poly <userlib>:"Build Path__ogtk.vi"("name or relative path"=w330, "base path"=w331) -> ("appended path"=w329:path[])
          n123 = for {
            tunnel: w329 -> [w337] mode=indexing
            tunnel: [w336] -> w326 mode=indexing if=w335
            tunnel: w321 -> [w333]
            tunnel: [w332] -> w328 mode=indexing
            n124 = call <vilib>:"Get File Extension.vi"("error in (no error)"=w333, "file"=w337) -> ("error out"=w332:errorcluster, "lowercase file extension"=w334:string, "dup file"=w336:path)  [unwired: 5 in, 2 out]
            n125 = Not Equal?(x=w334, y="ini") -> (x != y?=w335:bool)
          }
          n126 = Merge Errors(w328) -> (w327:errorcluster)
        }
        n127 = Bundle By Name(cluster=w311, "Files"=w313) -> (w312:T3)
        n128 = Merge Errors(w316) -> (w314:errorcluster)
        n129 = call <vilib>:"Add State(s) to Queue__jki_lib_state_machine.vi"("State(s) in (\"\")"=w319) -> ("States Out"=w318:string)  [unwired: 14 in]
      }
      frame "PGSQL: Get DSC Path" {
        # "Template Separator\n(You can make a copy of, or modify, this frame)"
        n130 = Unbundle By Name(w339) -> ("Files"=w346:path[][])
        n131 = Index Array(array=w346, index (col)=0 ("disabled index (col)")) -> (element=w344:path[])  [unwired: 1 in]
        n132 = for {
          tunnel: w344 -> [w351] mode=indexing
          tunnel: [w357] -> w342 mode=indexing if=w353
          tunnel: [w356] -> w343 mode=indexing if=w353
          tunnel: [w355] -> w341 mode=indexing if=w353
          n133 = Not A Number/Path/Refnum?(number/path/refnum=w351) -> (NaN/Path/Refnum?=w352:bool)
          n134 = case shown="False" w352 {
            tunnel: [w378 w379] -> w357
            tunnel: [w377 w379] -> w356
            tunnel: [w376 w379] -> w355
            tunnel: [w368 FALSE] -> w353
            tunnel: w351 -> [w366 _]
            frame False {
              n135 = Read from Text File(file (use dialog)=w366, count=1) -> (text=w364:string[], error out=w358:errorcluster)  [unwired: 2 in, 2 out]
              n136 = Index Array(array=w364) -> (element=w365:string)  [unwired: 1 in]
              n137 = Spreadsheet String To Array(format string="%s", spreadsheet string=w365, array type (2D Dbl)=w364) -> (array=w363:string[])  [unwired: 1 in]
              n138 = Index Array(array=w363, index=2) -> (element=w361:string)
              n139 = Match Pattern(string=w361, regular expression="\\\\\\\\housesoftheholy\\\\default_database\\\\HousesoftheHoly\\\\" ("delimiter")) -> (after substring=w374:string)  [unwired: 1 in, 3 out]
              n140 = Unbundle By Name(w358) -> ("status"=w369:bool)
              n141 = Match Pattern(string=w374, regular expression="\\\\") -> (before substring=w378:string, after substring=w372:string)  [unwired: 1 in, 2 out]
              n142 = Match Pattern(string=w372, regular expression=" (") -> (before substring=w377:string, after substring=w370:string)  [unwired: 1 in, 2 out]
              n143 = Not(x=w369) -> (.not. x?=w368:bool)
              n144 = Match Pattern(string=w370, regular expression=")") -> (before substring=w376:string)  [unwired: 1 in, 3 out]
            }
            frame True {
              w379 = ""
            }
          }
          n145 = Format Into String(format string="Listing %s", w351) -> (resulting string=w354:string)  [unwired: 2 in, 1 out]
          n146 = local write "Status"(w354) -> ()
        }
        n147 = Bundle By Name(cluster=w339, "DSC Table"=w342, "DSC Variable"=w343, "DSC Units"=w341) -> (w340:T3)
        n148 = call <vilib>:"Add State(s) to Queue__jki_lib_state_machine.vi"("State(s) in (\"\")"=w349) -> ("States Out"=w348:string)  [unwired: 14 in]
      }
      frame "PGSQL: Get PGSQL Path" {
        # "Template Separator\n(You can make a copy of, or modify, this frame)"
        n149 = Unbundle By Name(w386) -> ("DSC Table"=w389:string[], "DSC Variable"=w388:string[], "Data.PG"=w385:refnum<class "LV-Data.PGSQL.lvclass">)  [unwired: 1 out]
        n150 = for {
          tunnel: w389 -> [w404] mode=indexing
          tunnel: w388 -> [w411] mode=indexing
          tunnel: w384 -> [w410]
          tunnel: [w408] -> w383
          tunnel: [w406] -> w382 mode=indexing
          shift-right: [w407] -> w381
          shift-left: w385 -> [w409]
          n151 = call "List Tables.vi"("error in (no error)"=w410, "Data.PG"=w409) -> ("error out"=w400:errorcluster, "Table Names"=w417:string[], "Data.PG"=w414:refnum<class "LV-Data.PGSQL.lvclass">)  [unwired: 6 in, 1 out]
          n152 = call "Is Value Changed.vim"("value"=w404) -> ("changed or first call?"=w405:bool)
          n153 = feedback #1() -> (w403:string)  [unwired: 1 in]
          n154 = Select(t=w404, s=w405, f=w403) -> (s? t:f=w401:string)
          n155 = call "DSC TSV to PGSQL Choose Column Dialog.vi"("error in"=w400, "Message"="Choose Table", "DSC"=w401, "Item Names"=w417) -> ("error out"=w399:errorcluster, "Selection"=w402:string)  [unwired: 6 in]
          n156 = feedback-in #1(w402) -> ()
          n157 = call "Get Table Path.vi"("error in (no error)"=w399, "Table Name"=w402, "Data.PG"=w414) -> ("error out"=w412:errorcluster, "Table Path"=w393:string, "Data.PG out"=w413:refnum<class "LV-Data.PGSQL.lvclass">)  [unwired: 5 in, 1 out]
          n158 = call "List Columns.vi"("error in (no error)"=w412, "Table Path"=w393, "Data.PG"=w413) -> ("error out"=w398:errorcluster, "Column Names"=w416:string[], "Data.PG out"=w415:refnum<class "LV-Data.PGSQL.lvclass">)  [unwired: 4 in, 2 out]
          n159 = call "DSC TSV to PGSQL Choose Column Dialog.vi"("error in"=w398, "Message"="Choose Column", "DSC"=w411, "Item Names"=w416) -> ("error out"=w397:errorcluster, "Selection"=w394:string)  [unwired: 6 in]
          n160 = call "Get Column Path.vi"("error in (no error)"=w397, "Column Name"=w394, "Table path"=w393, "Data.PG in"=w415) -> ("error out"=w408:errorcluster, "Column Unit"=w395:string, "Column Path"=w418:string, "Data.PG out"=w407:refnum<class "LV-Data.PGSQL.lvclass">)  [unwired: 4 in]
          n161 = call "Build Path.vi"("Table path"=w393, "Column path"=w418, "Table name"=w402, "Column name"=w394, "Column units"=w395) -> ("PG path"=w406:string)  [unwired: 10 in]
        }
        n162 = Bundle By Name(cluster=w386, "PGSQL Paths"=w382, "Data.PG"=w381) -> (w387:T3)
        n163 = call <vilib>:"Add State(s) to Queue__jki_lib_state_machine.vi"("State(s) in (\"\")"=w391) -> ("States Out"=w390:string)  [unwired: 14 in]
      }
      frame "PGSQL: Process Files" {
        # "Template Separator\n(You can make a copy of, or modify, this frame)"
        n164 = Unbundle By Name(w428) -> ("Data.PG"=w421:refnum<class "LV-Data.PGSQL.lvclass">, "PGSQL Paths"=w420:string[], "Files"=w419:path[][])
        n165 = control-ref of="Status"() -> (w422:refnum<vi>)
        n166 = for {
          tunnel: w419 -> [w437] mode=indexing
          tunnel: w420 -> [w436] mode=indexing
          tunnel: w421 -> [w435]
          tunnel: w425 -> [w434]
          tunnel: [w433] -> w424
          tunnel: [w432] -> w423 mode=indexing
          tunnel: w422 -> [w431]
          # "Variable"
          n167 = for {
            tunnel: w437 -> [w438] mode=indexing
            tunnel: w436 -> [w439]
            tunnel: w435 -> [w440]
            tunnel: w434 -> [w442]
            tunnel: [w446] -> w433
            tunnel: [w443] -> w432 mode=indexing if=w444
            tunnel: w431 -> [w441]
            # "File (Year)"
            n168 = call "DSC TSV Process Files with Queues.vi"("reference"=w441, "error in"=w442, "File Path"=w438, "variable"=w439, "Data.PG in"=w440) -> ("error out"=w446:errorcluster)  [unwired: 6 in]
            n169 = Unbundle By Name(w446) -> ("status"=w445:bool)
            n170 = Path To String(path=w438) -> (string=w443:string)
            n171 = Not(x=w445) -> (.not. x?=w444:bool)
          }
        }
        n172 = Array To Spreadsheet String(array=w423, 3:"%s" ("format string")) -> (spreadsheet string=→"Processed Files":string)  [unwired: 1 in]
        n173 = call <vilib>:"Add State(s) to Queue__jki_lib_state_machine.vi"("State(s) in (\"\")"=w430) -> ("States Out"=w429:string)  [unwired: 14 in]
      }
    }
  }
